vi "A170316-11_Auto.vi"() -> ()   [LabVIEW 2020]
uses:
  Global_Variable/A170316-11.vi
  Global_Variable/Global.vi
  Database/Global1.vi
  <vilib>/addons/database/Connection.llb/DB Tools Open Connec (String).vi
  <vilib>/addons/database/NI_Database_API.lvlib
panel:
  out "请再次确认扭矩":bool
  in  "更换产品":refnum<vi>
  out "刻线涂色标":bool
  out "涂下传动轴螺栓色标":bool
  out "拆下辅具安装下轴固定螺栓并确认扭矩":bool
  in  "前序OK？":string
  out "主观判断是否合格":bool
  out "右转两圈检测":bool
  out "左转两圈检测":bool
  out "按启动按钮":bool
  out "涂下轴固定螺栓色标":bool
  out "安装下传动轴辅具螺栓并确认扭矩":bool
  out "请扫码":bool
  out "磨合次数":i32
  in  "判定结果":bool[][](array[boolean])=[[TRUE]]
  in  "STEP":string
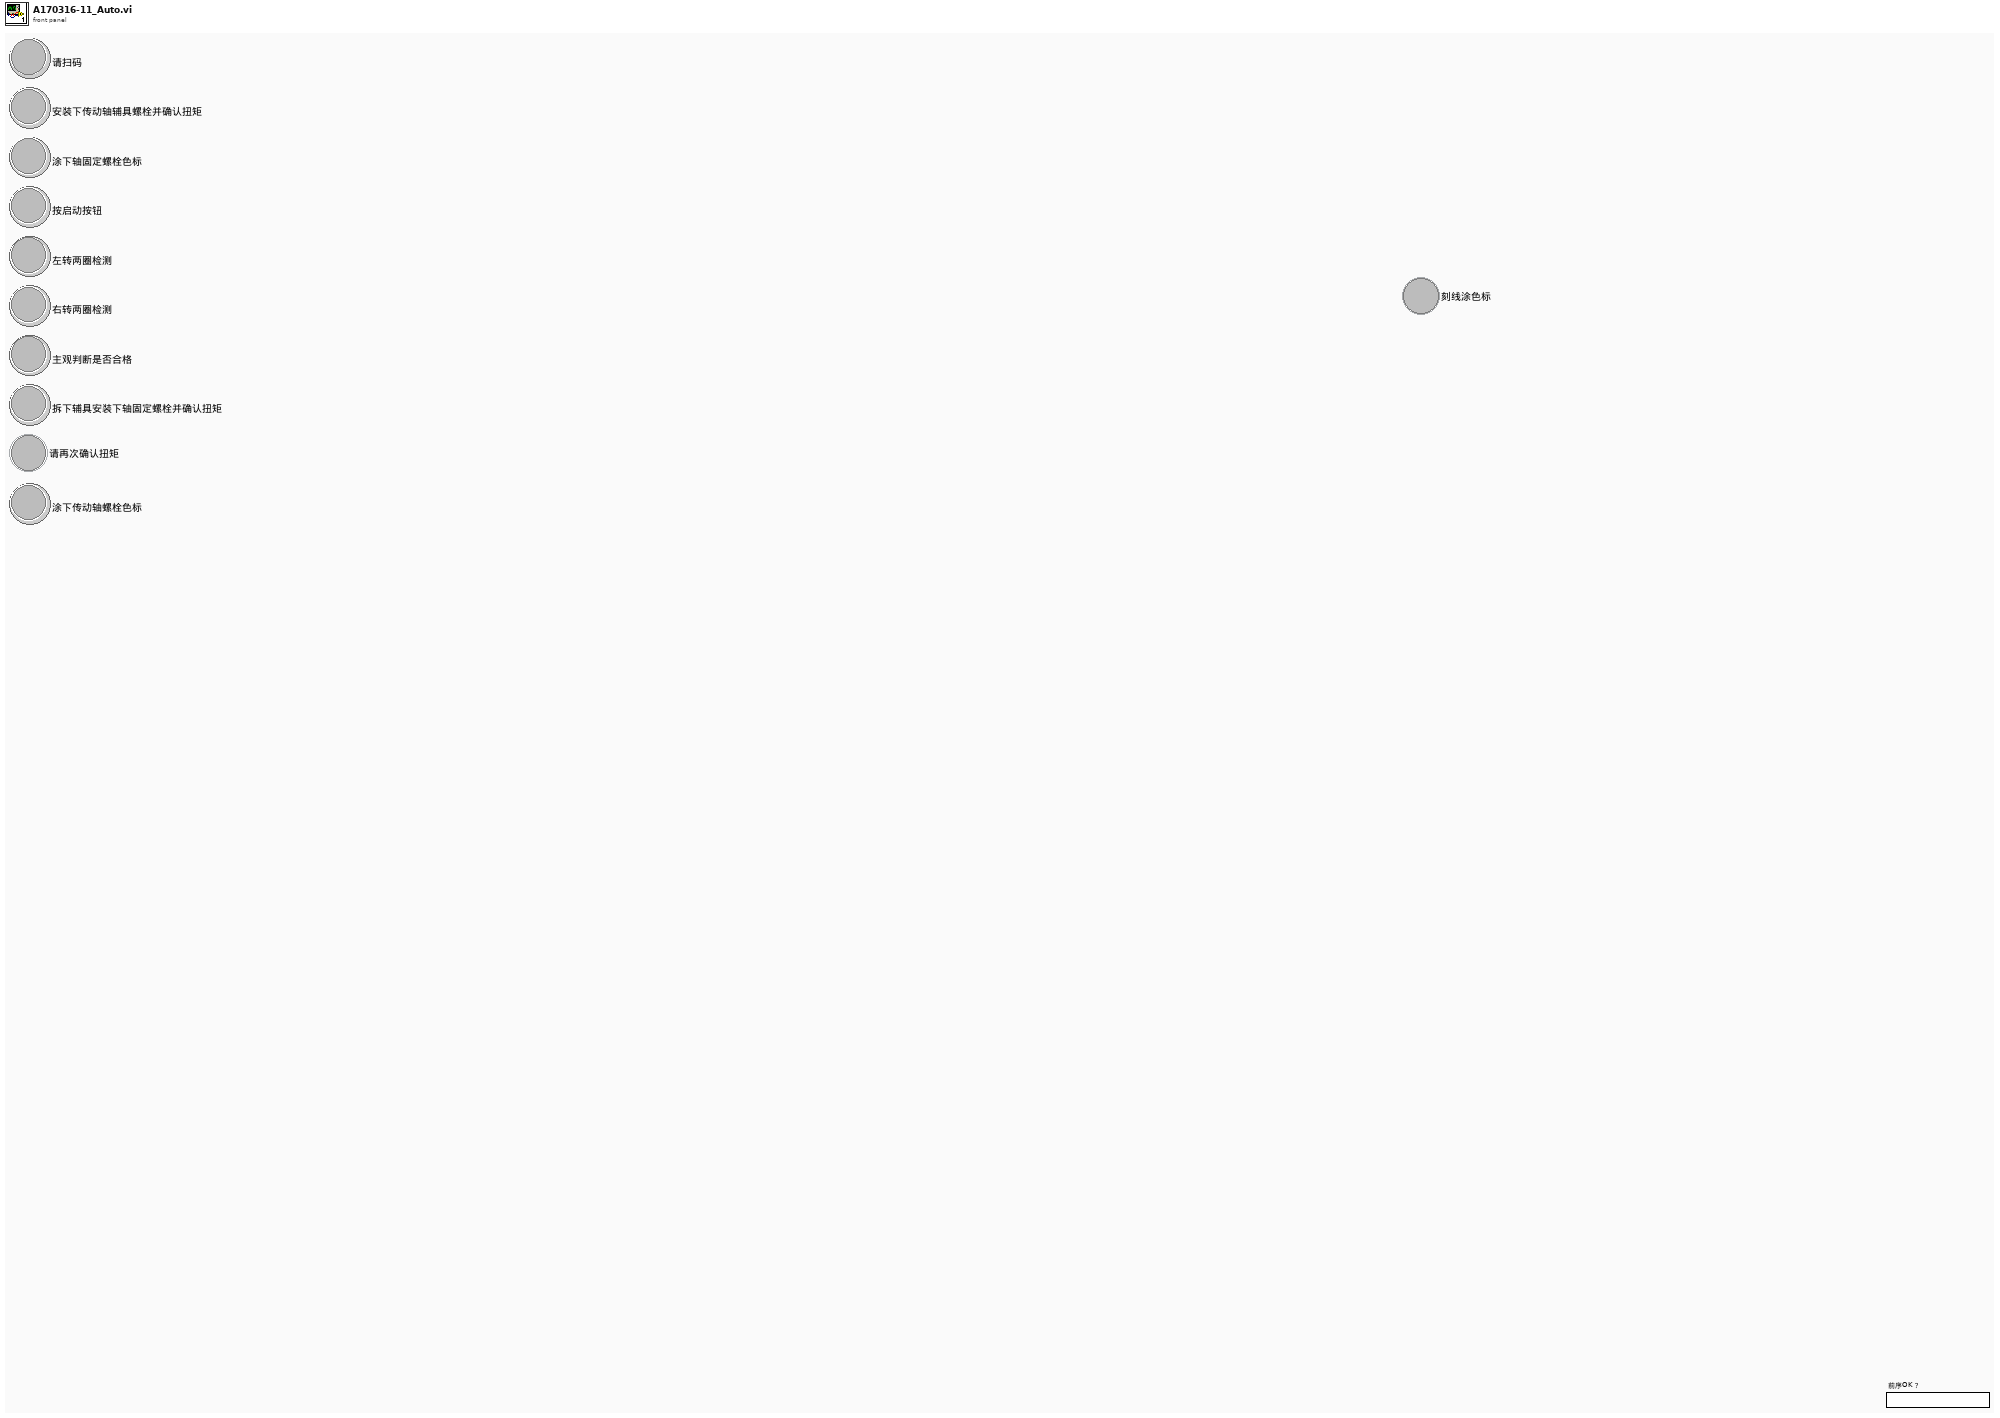
[diagram p1: front panel]
types:
  T1 = typedef "NI_Database_API.lvlib/Conn ObjectReference.ctl" = refnum<k1>
  T2 = cluster{i64, i64, i64, "生产结果":string, "result string":string}
  T3 = cluster{i64, i64, i64, "生产结果":string, "result string":string}[]
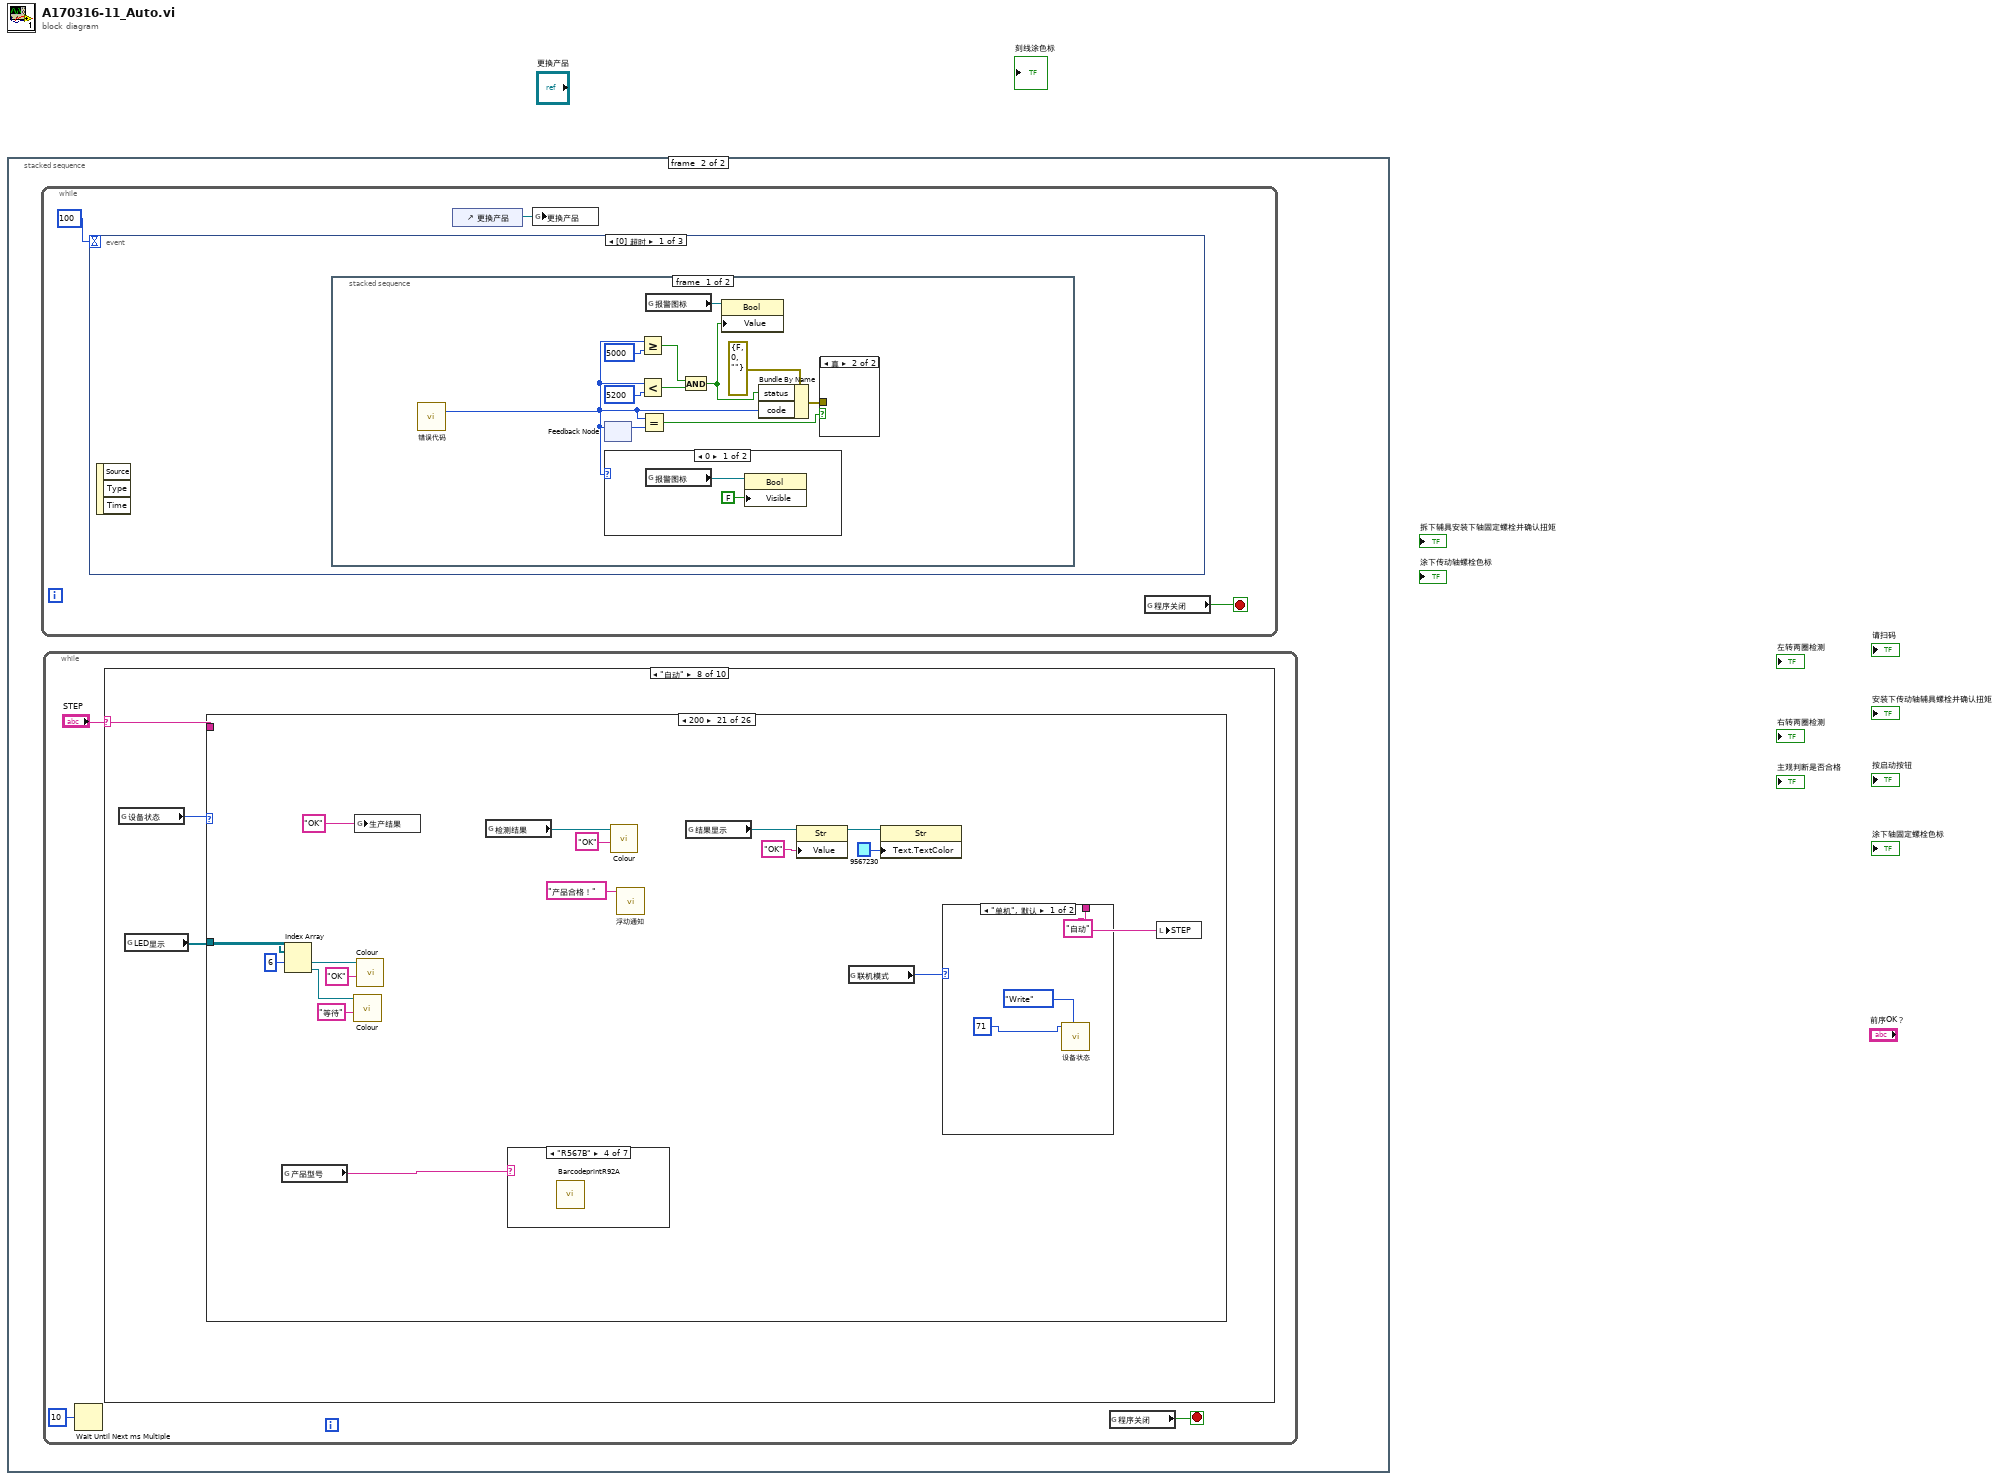
[diagram p0: block diagram]
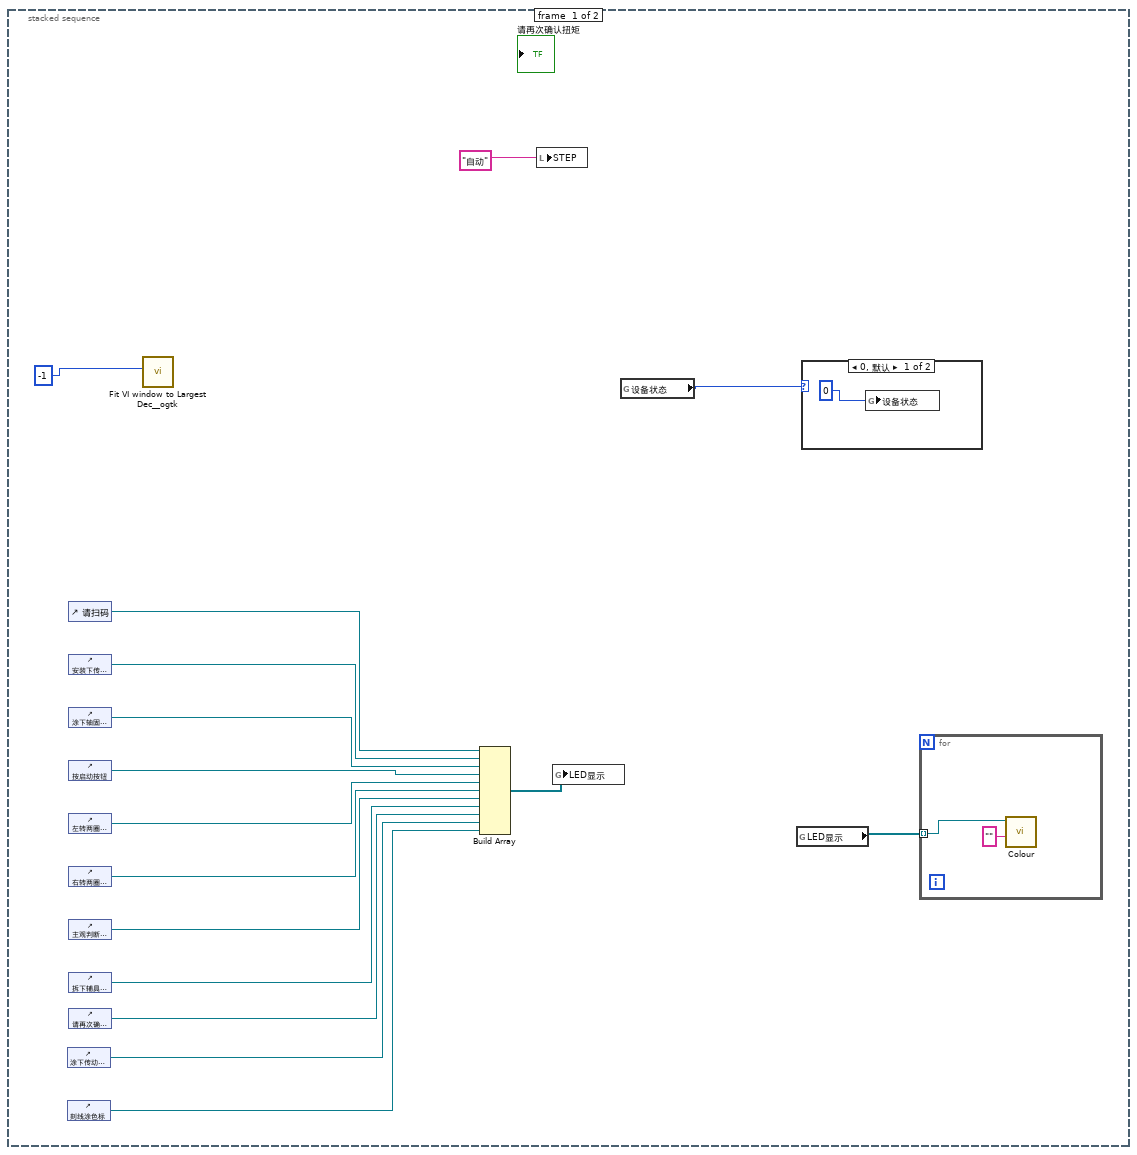
[diagram p2: hidden frame]
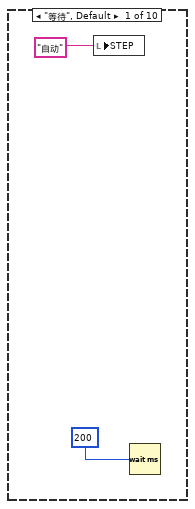
[diagram p4: hidden frame]
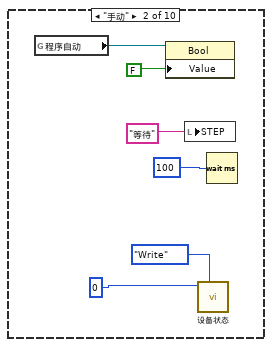
[diagram p5: hidden frame]
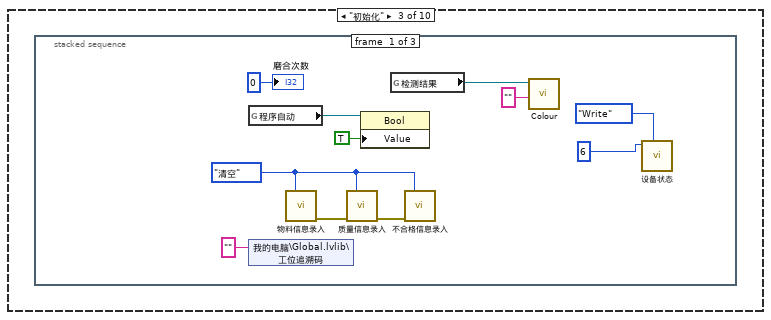
[diagram p6: hidden frame]
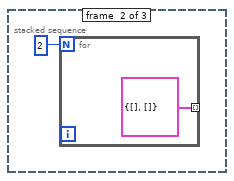
[diagram p7: hidden frame]
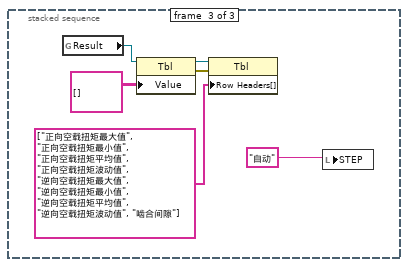
[diagram p8: hidden frame]
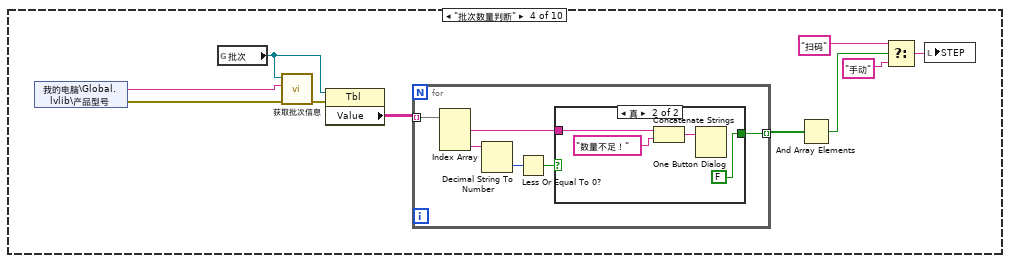
[diagram p9: hidden frame]
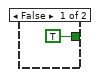
[diagram p10: hidden frame]
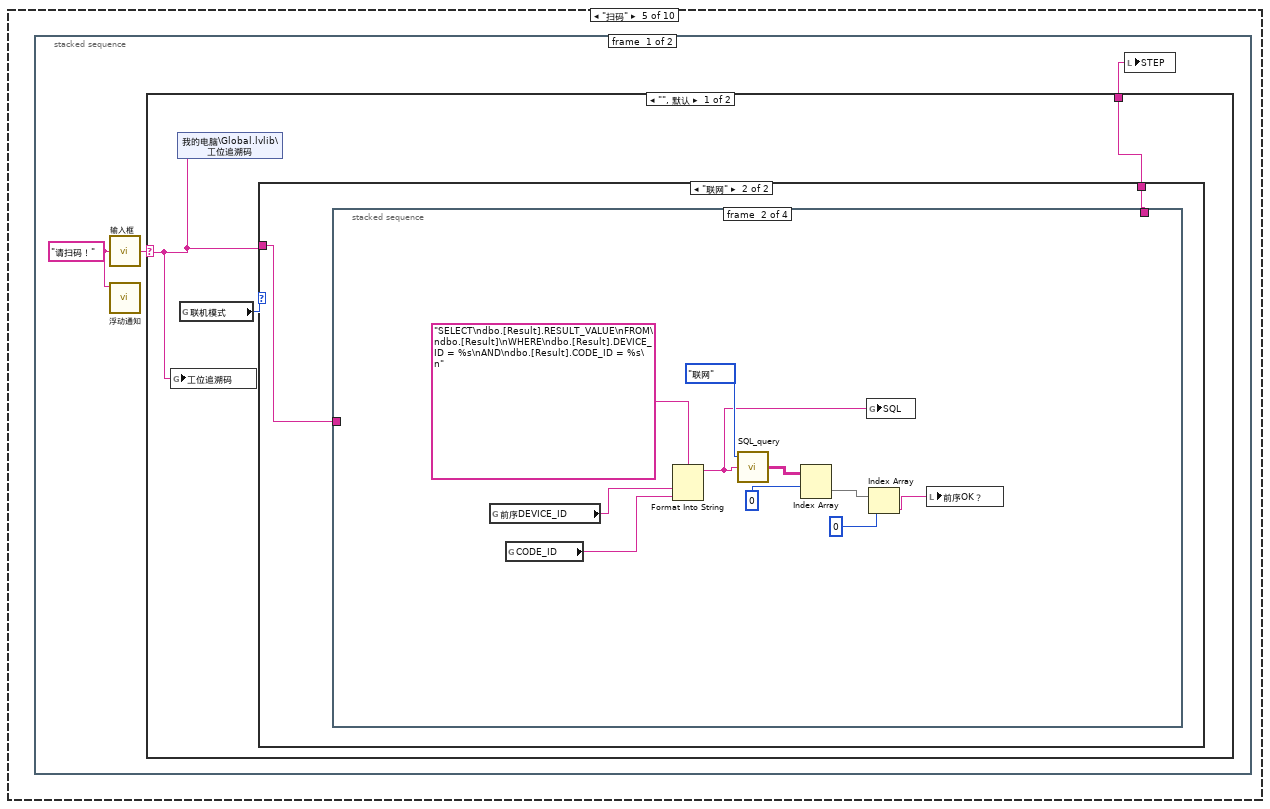
[diagram p11: hidden frame]
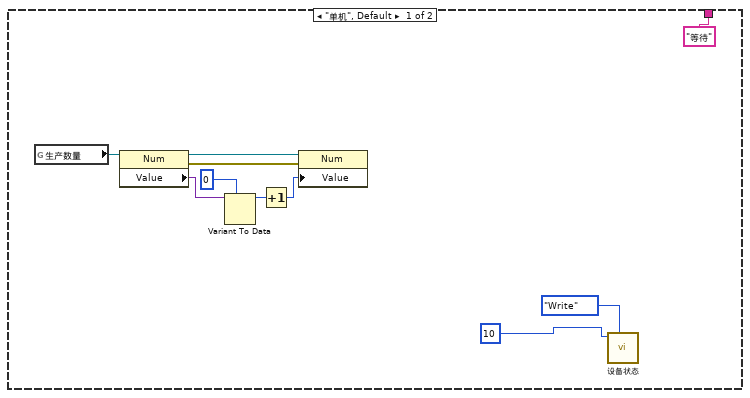
[diagram p12: hidden frame]
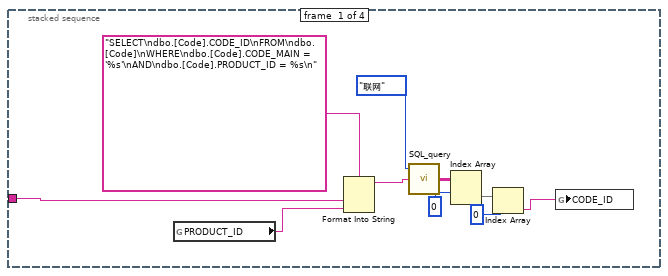
[diagram p13: hidden frame]
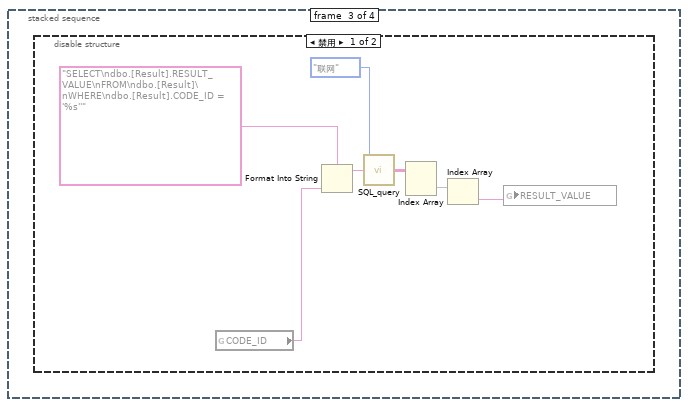
[diagram p14: hidden frame]
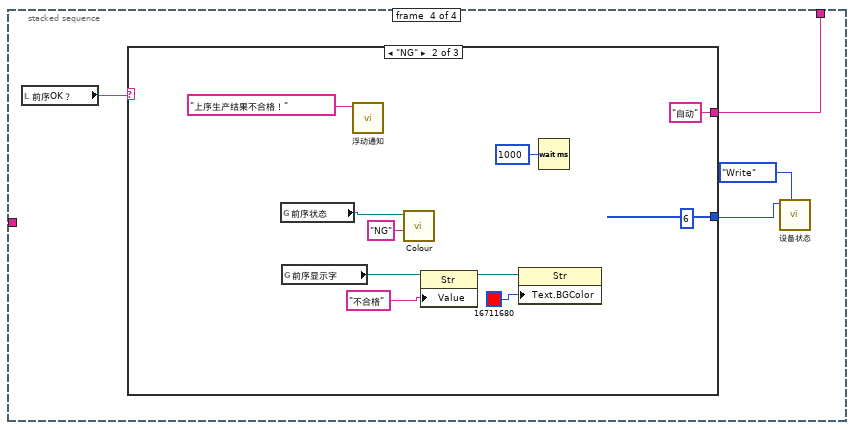
[diagram p16: hidden frame]
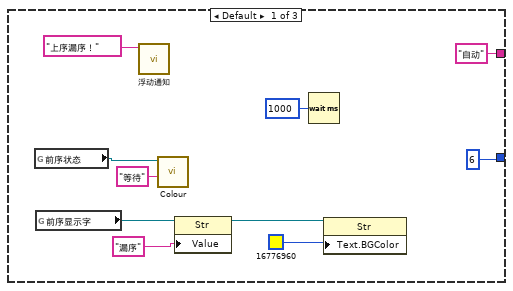
[diagram p17: hidden frame]
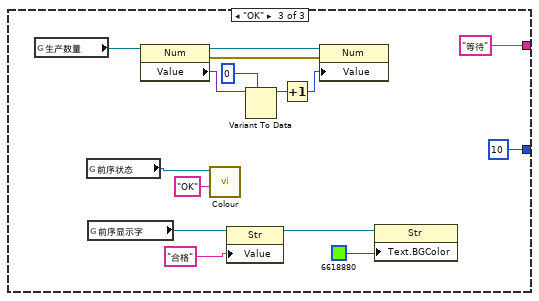
[diagram p18: hidden frame]
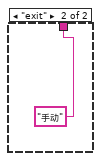
[diagram p19: hidden frame]
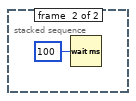
[diagram p20: hidden frame]
diagram:
  n1 = stacked-sequence {
    frame #0 {
      n2 = control-ref of="涂下传动轴螺栓色标"() -> (w4:refnum<vi>)
      n3 = control-ref of="刻线涂色标"() -> (w3:refnum<vi>)
      n4 = control-ref of="请扫码"() -> (w14:refnum<vi>)
      n5 = control-ref of="安装下传动轴辅具螺栓并确认扭矩"() -> (w13:refnum<vi>)
      n6 = control-ref of="涂下轴固定螺栓色标"() -> (w12:refnum<vi>)
      n7 = control-ref of="按启动按钮"() -> (w11:refnum<vi>)
      n8 = control-ref of="左转两圈检测"() -> (w10:refnum<vi>)
      n9 = control-ref of="右转两圈检测"() -> (w9:refnum<vi>)
      n10 = control-ref of="主观判断是否合格"() -> (w8:refnum<vi>)
      n11 = control-ref of="拆下辅具安装下轴固定螺栓并确认扭矩"() -> (w5:refnum<vi>)
      n12 = control-ref of="请再次确认扭矩"() -> (w2:refnum<vi>)
      n13 = call <userlib>:"Fit VI window to Largest Dec__ogtk.vi"("border spacing (2 px)"=-1) -> ()  [unwired: 5 in, 2 out]
      n14 = Build Array(w14, w13, w12, w11, w10, w9, w8, w5, w2, w4, w3) -> (w7:refnum<vi>[])
      n15 = local write "STEP"("自动" ("STEP")) -> ()
      n16 = global write "A170316-11.vi" "LED显示"(w7) -> ()
      n17 = global read "Global.vi" "设备状态"() -> (w1:i32)
      n18 = global read "A170316-11.vi" "LED显示"() -> (w6:refnum<vi>[])
      n19 = case shown="0, 默认" w1 {
        frame 0, Default {
          n20 = global write "Global.vi" "设备状态"(i16 0 ("设备状态")) -> ()
        }
        frame 3721..3723 {
        }
      }
      n21 = for {
        tunnel: w6 -> [w19] mode=indexing
        n22 = call "Colour.vi"("result"="", "colourRef"=w19) -> ()  [unwired: 9 in, 1 out]
      }
    }
    frame #1 {
      n23 = while {
        stop <- w463 stop-if-true
        n24 = event shown="[0] 超时" {
          selector: _ -> [_ _ _]
          dyn-events: _ -> [_ _ _]
          timeout: 100 -> [_ _ _]
          event Timeout {
            n25 = event-data() -> ()  [unwired: 1 in, 3 out]
            n26 = stacked-sequence {
              frame #0 {
                n27 = call "错误代码.vi"() -> ("Status_Read"=w465:u32)  [unwired: 11 in]
                n28 = feedback #1() -> (w475:u32)  [unwired: 1 in]
                n29 = feedback-in #1(w465) -> ()
                n30 = case shown="0" w465 {
                  frame 0 {
                    n31 = global read "Global.vi" "报警图标"() -> (w476:refnum<vi>)
                    n32 = property class="Bool"(reference=w476, "Visible"=FALSE ("可见")) -> ()  [unwired: 1 in, 2 out]
                  }
                  frame 1, Default {
                    n33 = global read "Global.vi" "报警图标"() -> (w479:refnum<vi>)
                    n34 = property class="Bool"(reference=w479, "Visible"=TRUE ("可见")) -> ()  [unwired: 1 in, 2 out]
                  }
                }
                n35 = Greater Or Equal?(x=w465, y=i16 5000) -> (x >= y?=w473:bool)
                n36 = Less?(x=w465, y=i16 5200) -> (x < y?=w474:bool)
                n37 = Equal?(x=w465, y=w475) -> (x = y?=w472:bool)
                n38 = global read "Global.vi" "报警图标"() -> (w467:refnum<vi>)
                n39 = And(x=w473, y=w474) -> (x .and. y?=w466:bool)
                n40 = property class="Bool"(reference=w467, "Value"=w466) -> ()  [unwired: 1 in, 2 out]
                n41 = Bundle By Name(cluster=errorcluster {"status"=FALSE, "code"=0, "source"=""} ("错误常量"), "status"=w466, "code"=w465) -> (w471:errorcluster)
                n42 = case shown="真" w472 {
                  tunnel: w471 -> [w480 _]
                  frame False {
                    n43 = call "报警处理.vi"("错误常量"=w480) -> ()  [unwired: 9 in, 2 out]
                  }
                  frame True {
                  }
                }
              }
              frame #1 {
                n44 = disable-structure shown="禁用" {
                  frame Disabled {
                    n45 = global read "Global.vi" "程序自动"() -> (w484:refnum<vi>)
                    n46 = property class="Bool"(reference=w484) -> ("Value"=w483:variant)  [unwired: 1 in, 2 out]
                    n47 = Variant To Data(type=FALSE, Variant=w483) -> (data=w481:bool)  [unwired: 1 in, 1 out]
                    n48 = case shown="真" w481 {
                      selector: w481 -> [w486 _]
                      frame False {
                        n49 = call <userlib>:"Boolean Trigger__ogtk.vi"("Boolean Input"=w486) -> ("Rising Edge"=w485:bool)  [unwired: 1 in, 1 out]
                        n50 = case shown="真" w485 {
                          frame False {
                          }
                          frame True {
                            n51 = local write "STEP"("手动" ("STEP")) -> ()
                          }
                        }
                      }
                      frame True {
                        n52 = shared-variable "我的电脑\\A17031611.lvlib\\设备状态"() -> (w488:i16)  [unwired: 1 in, 1 out]
                        n53 = case shown="5" w488 {
                          frame 0, Default {
                            n54 = global read "Global.vi" "程序自动"() -> (w490:refnum<vi>)
                            n55 = call "浮动通知.vi"("通知内容"="请复位") -> ()  [unwired: 11 in]
                            n56 = property class="Bool"(reference=w490, "Value"=FALSE) -> ()  [unwired: 1 in, 2 out]
                          }
                          frame 5 {
                            n57 = local write "STEP"("初始化" ("STEP")) -> ()
                          }
                        }
                      }
                    }
                  }
                  frame Enabled {
                  }
                }
              }
            }
          }
          event "更换产品": Value Change {
            n58 = event-data() -> ()  [unwired: 1 in, 6 out]
            n59 = global read "A170316-11.vi" "LED显示"() -> (w495:refnum<vi>[])
            n60 = global read "Global.vi" "操作步骤"() -> (w493:bool[])
            n61 = for "For循环" {
              tunnel: w493 -> [w499] mode=indexing
              tunnel: w495 -> [w498] mode=indexing
              shift-right: [w496] -> _
              shift-left: 360 -> [w497]
              n62 = case shown="真" w499 {
                tunnel: w498 -> [w501 w503]
                tunnel: w497 -> [w502 w508]
                tunnel: [w502 w505] -> w496
                frame False {
                  n63 = property class="Bool (严格)"(reference=w501, "Top"=-100 ("位置:置顶")) -> ()  [unwired: 1 in, 2 out]
                }
                frame True {
                  n64 = Add(x=w508, y=65) -> (x+y=w505:i32)
                  n65 = Bundle(-1510, w505) -> (w506:cluster{i32, i32})  [unwired: 1 in]
                  n66 = property class="Bool (严格)"(reference=w503, "Position"=w506) -> ()  [unwired: 1 in, 2 out]
                }
              }
            }
          }
          event Panel Close {
            n67 = event-data() -> ()  [unwired: 1 in, 4 out]
            n68 = global write "Global.vi" "程序关闭"(TRUE ("程序关闭")) -> ()
          }
        }
        n69 = control-ref of="更换产品"() -> (w462:refnum<vi>)
        n70 = global write "Global.vi" "更换产品"(w462) -> ()
        n71 = global read "Global.vi" "程序关闭"() -> (w463:bool)
      }
      n72 = while {
        stop <- w21 stop-if-true
        n73 = Wait Until Next ms Multiple(millisecond multiple=u32 10 ("毫秒倍数")) -> ()  [unwired: 1 out]
        n74 = case shown="\"自动\"" "STEP" {
          selector: "STEP" -> [_ _ _ _ _ _ _ w248 _ _]
          frame "等待", Default {
            n75 = local write "STEP"("自动" ("STEP")) -> ()
            n76 = Wait (ms)(milliseconds to wait=u32 200 ("等待时间（毫秒）")) -> ()  [unwired: 1 out]
          }
          frame "手动" {
            n77 = global read "Global.vi" "程序自动"() -> (w28:refnum<vi>)
            n78 = property class="Bool"(reference=w28, "Value"=FALSE) -> ()  [unwired: 1 in, 2 out]
            n79 = local write "STEP"("等待" ("STEP")) -> ()
            n80 = call "设备状态.vi"("枚举"=enum16{"Read", "Write"}."Write", "Status_Write"=u16 0 ("设备状态")) -> ()  [unwired: 9 in, 1 out]
            n81 = Wait (ms)(milliseconds to wait=u32 100 ("等待时间（毫秒）")) -> ()  [unwired: 1 out]
          }
          frame "初始化" {
            n82 = stacked-sequence {
              frame #0 {
                w40 = enum16{"录入", "清空"}."清空" ("功能")
                n83 = global read "Global.vi" "程序自动"() -> (w36:refnum<vi>)
                n84 = shared-variable "我的电脑\\Global.lvlib\\工位追溯码"("" ("传感器码")) -> ()  [unwired: 1 in, 1 out]
                n85 = call "物料信息录入.vi"("功能"=w40) -> ("错误输出"=w39:errorcluster)  [unwired: 14 in]
                n86 = call "质量信息录入.vi"("功能"=w40, "错误输入（无错误）"=w39) -> ("错误输出"=w41:errorcluster)  [unwired: 13 in]
                n87 = property class="Bool"(reference=w36, "Value"=TRUE) -> ()  [unwired: 1 in, 2 out]
                n88 = global read "Global.vi" "检测结果"() -> (w34:refnum<vi>)
                n89 = call "不合格信息录入.vi"("功能"=w40, "错误输入（无错误）"=w41) -> ()  [unwired: 13 in, 1 out]
                n90 = call "Colour.vi"("result"="", "colourRef"=w34) -> ()  [unwired: 9 in, 1 out]
                n91 = call "设备状态.vi"("枚举"=enum16{"Read", "Write"}."Write", "Status_Write"=i16 6 ("设备状态")) -> ()  [unwired: 9 in, 1 out]
                "磨合次数" <- 0 ("磨合次数")
              }
              frame #1 {
                n92 = for {
                  N: 2 -> [_]
                  tunnel: [cluster{dbl[], dbl[]} {[], []}] -> _ mode=indexing
                }
              }
              frame #2 {
                n93 = global read "Global.vi" "Result"() -> (w47:refnum<vi>)
                n94 = property class="Tbl"(reference=w47, "Value"=string[][] []) -> (reference out=w48:refnum<vi>, error out=w49:errorcluster)  [unwired: 1 in]
                n95 = property class="Tbl"(reference=w48, error in=w49, "Row Headers[]"=string[] ["正向空载扭矩最大值", "正向空载扭矩最小值", "正向空载扭矩平均值", "正向空载扭矩波动值", "逆向空载扭矩最大值", "逆向空载扭矩最小值", "逆向空载扭矩平均值", "逆向空载扭矩波动值", "啮合间隙"] ("列首字符串[]")) -> ()  [unwired: 2 out]
                n96 = local write "STEP"("自动" ("result")) -> ()
              }
            }
          }
          frame "批次数量判断" {
            n97 = shared-variable "我的电脑\\Global.lvlib\\产品型号"() -> (w55:string, error out=w58:errorcluster)  [unwired: 1 in]
            n98 = global read "Global.vi" "批次"() -> (w56:refnum<vi>)
            n99 = call "获取批次信息.vi"("error in (no error)"=w58, "产品型号"=w55, "Tbl引用句柄"=w56) -> ("error out"=w57:errorcluster)  [unwired: 7 in, 1 out]
            n100 = property class="Tbl"(reference=w56, error in=w57) -> ("Value"=w59:string[][])  [unwired: 2 out]
            n101 = for {
              tunnel: w59 -> [w65] mode=indexing
              tunnel: [w60] -> w54 mode=indexing
              n102 = Index Array(array=w65) -> (element #1=w61:string, element #3=w64:string)  [unwired: 3 in, 1 out]
              n103 = Decimal String To Number(string=w64) -> (number=w63:i32)  [unwired: 2 in, 1 out]
              n104 = Less Or Equal To 0?(x=w63) -> (x <= 0?=w62:bool)
              n105 = case shown="真" w62 {
                tunnel: w61 -> [_ w70]
                tunnel: [TRUE FALSE] -> w60
                frame False {
                }
                frame True {
                  n106 = Concatenate Strings(w70, "数量不足！" ("字符串")) -> (w68:string)
                  n107 = One Button Dialog(message=w68) -> ()  [unwired: 1 in, 1 out]
                }
              }
            }
            n108 = And Array Elements(Boolean array=w54) -> (logical AND=w53:bool)
            n109 = Select(t="扫码" ("STEP"), s=w53, f="手动" ("STEP")) -> (s? t:f=w50:string)
            n110 = local write "STEP"(w50) -> ()
          }
          frame "扫码" {
            n111 = stacked-sequence {
              frame #0 {
                w72 = "请扫码！" ("提示信息")
                n112 = call "输入框.vi"("提示信息"=w72) -> ("条形码输出"=w73:string)
                n113 = call "浮动通知.vi"("通知内容"=w72) -> ()  [unwired: 11 in]
                n114 = case shown="\"\", 默认" w73 {
                  selector: w73 -> [w74 _]
                  tunnel: [w75 "手动"] -> w71
                  frame "", Default {
                    n115 = global write "Global1.vi" "工位追溯码"(w74) -> ()
                    n116 = shared-variable "我的电脑\\Global.lvlib\\工位追溯码"(w74) -> ()  [unwired: 1 in, 1 out]
                    n117 = global read "Global1.vi" "联机模式"() -> (w76:enum16{"单机", "联网"})
                    n118 = case shown="\"联网\"" w76 {
                      tunnel: w74 -> [_ w87]
                      tunnel: ["等待" w88] -> w75
                      frame "单机", Default {
                        n119 = global read "Global.vi" "生产数量"() -> (w81:refnum<vi>)
                        n120 = property class="Num"(reference=w81) -> (reference out=w82:refnum<vi>, error out=w83:errorcluster, "Value"=w84:variant)  [unwired: 1 in]
                        n121 = Variant To Data(type=u32 0, Variant=w84) -> (data=w85:u32)  [unwired: 1 in, 1 out]
                        n122 = Increment(x=w85) -> (x+1=w86:u32)
                        n123 = property class="Num"(reference=w82, error in=w83, "Value"=w86) -> ()  [unwired: 2 out]
                        n124 = call "设备状态.vi"("枚举"=enum16{"Read", "Write"}."Write", "Status_Write"=i16 10 ("设备状态控制字")) -> ()  [unwired: 9 in, 1 out]
                      }
                      frame "联网" {
                        n125 = stacked-sequence {
                          tunnel: w87 -> [w95 _ _ _]
                          tunnel: [_ _ _ w119] -> w88
                          frame #0 {
                            n126 = global read "Global1.vi" "PRODUCT_ID"() -> (w92:string)
                            n127 = Format Into String(format string="SELECT\ndbo.[Code].CODE_ID\nFROM\ndbo.[Code]\nWHERE\ndbo.[Code].CODE_MAIN = '%s'\nAND\ndbo.[Code].PRODUCT_ID = %s\n" ("格式字符串"), w95, w92) -> (resulting string=w94:string)  [unwired: 2 in, 1 out]
                            n128 = call "SQL_query.vi"("SQL query"=w94, "联机模式"=enum16{"单机", "联网"}."联网") -> ("data"=w98:string[][])  [unwired: 1 in, 2 out]
                            n129 = Index Array(array=w98, index (row)=0 ("索引 (行)")) -> (element=w97:string[])  [unwired: 1 in]
                            n130 = Index Array(array=w97, index=0 ("索引")) -> (element=w89:string)
                            n131 = global write "Global1.vi" "CODE_ID"(w89) -> ()
                          }
                          frame #1 {
                            n132 = global read "Global1.vi" "前序DEVICE_ID"() -> (w102:string)
                            n133 = global read "Global1.vi" "CODE_ID"() -> (w103:string)
                            n134 = Format Into String(format string="SELECT\ndbo.[Result].RESULT_VALUE\nFROM\ndbo.[Result]\nWHERE\ndbo.[Result].DEVICE_ID = %s\nAND\ndbo.[Result].CODE_ID = %s\n" ("格式字符串"), w102, w103) -> (resulting string=w99:string)  [unwired: 2 in, 1 out]
                            n135 = call "SQL_query.vi"("SQL query"=w99, "联机模式"=enum16{"单机", "联网"}."联网") -> ("data"=w108:string[][])  [unwired: 1 in, 2 out]
                            n136 = Index Array(array=w108, index (row)=0 ("索引 (行)")) -> (element=w100:string[])  [unwired: 1 in]
                            n137 = global write "Global1.vi" "SQL"(w99) -> ()
                            n138 = Index Array(array=w100, index=0 ("索引")) -> (element=w104:string)
                            n139 = local write "前序OK？"(w104) -> ()
                          }
                          frame #2 {
                            n140 = disable-structure shown="禁用" {
                              frame Disabled {
                                n141 = global read "Global1.vi" "CODE_ID"() -> (w110:string)
                                n142 = Format Into String(format string="SELECT\ndbo.[Result].RESULT_VALUE\nFROM\ndbo.[Result]\nWHERE\ndbo.[Result].CODE_ID = '%s''" ("格式字符串"), w110) -> (resulting string=w112:string)  [unwired: 2 in, 1 out]
                                n143 = call "SQL_query.vi"("SQL query"=w112, "联机模式"=enum16{"单机", "联网"}."联网") -> ("data"=w115:string[][])  [unwired: 1 in, 2 out]
                                n144 = Index Array(array=w115) -> (element=w113:string[])  [unwired: 2 in]
                                n145 = Index Array(array=w113) -> (element=w114:string)  [unwired: 1 in]
                                n146 = global write "Global1.vi" "RESULT_VALUE"(w114) -> ()
                              }
                              frame Enabled {
                              }
                            }
                          }
                          frame #3 {
                            n147 = local read "前序OK？"() -> (w118:string)
                            n148 = case shown="\"NG\"" w118 {
                              tunnel: [i16 6 ("设备状态控制字") i16 6 ("设备状态控制字") i16 10 ("设备状态控制字")] -> w117
                              tunnel: ["自动" "自动" "等待"] -> w119
                              frame Default {
                                n149 = global read "Global.vi" "前序状态"() -> (w125:refnum<vi>)
                                n150 = global read "Global.vi" "前序显示字"() -> (w126:refnum<vi>)
                                n151 = call "浮动通知.vi"("通知内容"="上序漏序！" ("Status")) -> ()  [unwired: 11 in]
                                n152 = call "Colour.vi"("result"="等待", "colourRef"=w125) -> ()  [unwired: 9 in, 1 out]
                                n153 = property class="Str"(reference=w126, "Value"="漏序" ("值")) -> (reference out=w122:refnum<vi>)  [unwired: 1 in, 1 out]
                                n154 = Wait (ms)(milliseconds to wait=u32 1000 ("等待时间（毫秒）")) -> ()  [unwired: 1 out]
                                n155 = property class="Str"(reference=w122, "Text.BGColor"=u32 16776960) -> ()  [unwired: 1 in, 2 out]
                              }
                              frame "NG" {
                                n156 = global read "Global.vi" "前序状态"() -> (w135:refnum<vi>)
                                n157 = global read "Global.vi" "前序显示字"() -> (w136:refnum<vi>)
                                n158 = call "浮动通知.vi"("通知内容"="上序生产结果不合格！" ("Status")) -> ()  [unwired: 11 in]
                                n159 = call "Colour.vi"("result"="NG", "colourRef"=w135) -> ()  [unwired: 9 in, 1 out]
                                n160 = property class="Str"(reference=w136, "Value"="不合格" ("值")) -> (reference out=w132:refnum<vi>)  [unwired: 1 in, 1 out]
                                n161 = property class="Str"(reference=w132, "Text.BGColor"=u32 16711680) -> ()  [unwired: 1 in, 2 out]
                                n162 = Wait (ms)(milliseconds to wait=u32 1000 ("等待时间（毫秒）")) -> ()  [unwired: 1 out]
                              }
                              frame "OK" {
                                n163 = global read "Global.vi" "生产数量"() -> (w152:refnum<vi>)
                                n164 = global read "Global.vi" "前序状态"() -> (w144:refnum<vi>)
                                n165 = global read "Global.vi" "前序显示字"() -> (w145:refnum<vi>)
                                n166 = property class="Num"(reference=w152) -> (reference out=w153:refnum<vi>, error out=w151:errorcluster, "Value"=w150:variant)  [unwired: 1 in]
                                n167 = call "Colour.vi"("result"="OK", "colourRef"=w144) -> ()  [unwired: 9 in, 1 out]
                                n168 = property class="Str"(reference=w145, "Value"="合格" ("值")) -> (reference out=w141:refnum<vi>)  [unwired: 1 in, 1 out]
                                n169 = Variant To Data(type=u32 0, Variant=w150) -> (data=w149:u32)  [unwired: 1 in, 1 out]
                                n170 = Increment(x=w149) -> (x+1=w148:u32)
                                n171 = property class="Num"(reference=w153, error in=w151, "Value"=w148) -> ()  [unwired: 2 out]
                                n172 = property class="Str"(reference=w141, "Text.BGColor"=u32 6618880) -> ()  [unwired: 1 in, 2 out]
                              }
                            }
                            n173 = call "设备状态.vi"("枚举"=enum16{"Read", "Write"}."Write", "Status_Write"=w117) -> ()  [unwired: 9 in, 1 out]
                          }
                        }
                      }
                    }
                  }
                  frame "exit" {
                  }
                }
                n174 = local write "STEP"(w71) -> ()
              }
              frame #1 {
                n175 = Wait (ms)(milliseconds to wait=u32 100 ("等待时间（毫秒）")) -> ()  [unwired: 1 out]
              }
            }
          }
          frame "录入数据库" {
            n176 = stacked-sequence {
              frame #0 {
                n177 = shared-variable "我的电脑\\Global.lvlib\\工位追溯码"() -> ()  [unwired: 1 in, 2 out]
                n178 = global read "Global1.vi" "工位追溯码"() -> (w157:string)
                n179 = global read "Global1.vi" "PRODUCT_ID"() -> (w161:string)
                n180 = Format Into String(format string="SELECT\ndbo.[Code].CODE_ID\nFROM\ndbo.[Code]\nWHERE\ndbo.[Code].CODE_MAIN = '%s'\nAND\ndbo.[Code].PRODUCT_ID = %s\n" ("格式字符串"), w157, w161) -> (resulting string=w163:string)  [unwired: 2 in, 1 out]
                n181 = call "SQL_query.vi"("SQL query"=w163, "联机模式"=enum16{"单机", "联网"}."联网") -> ("data"=w166:string[][])  [unwired: 1 in, 2 out]
                n182 = Index Array(array=w166, index (row)=0 ("索引 (行)")) -> (element=w165:string[])  [unwired: 1 in]
                n183 = Index Array(array=w165, index=0 ("索引")) -> (element=w158:string)
                n184 = global write "Global1.vi" "CODE_ID"(w158) -> ()
              }
              frame #1 {
                n185 = global read "Global1.vi" "CODE_ID"() -> (w168:string)
                n186 = Format Into String(format string="SELECT\ndbo.[Result].RESULT_VALUE\nFROM\ndbo.[Result]\nWHERE\ndbo.[Result].CODE_ID = %s" ("格式字符串"), w168) -> (resulting string=w170:string)  [unwired: 2 in, 1 out]
                n187 = call "SQL_query.vi"("SQL query"=w170, "联机模式"=enum16{"单机", "联网"}."联网") -> ("data"=w172:string[][])  [unwired: 1 in, 2 out]
                n188 = Index Array(array=w172) -> (element=w171:string[])  [unwired: 2 in]
                n189 = Index Array(array=w171) -> ()  [unwired: 1 in, 1 out]
              }
              frame #2 {
                n190 = Get Date/Time String(date format (0)=enum16{"short", "long", "abbreviated"}."short" ("日期格式(0)"), want seconds? (F)=FALSE ("需要秒？(F)")) -> (date string=w182:string, time string=w183:string)  [unwired: 1 in]
                n191 = global read "Global1.vi" "DEVICE_ID"() -> (w186:string)
                n192 = global read "Global1.vi" "USER_ID"() -> (w184:string)
                n193 = global read "Global1.vi" "CODE_ID"() -> (w185:string)
                n194 = global read "Global1.vi" "生产结果"() -> (w177:string)
                n195 = global read "Global1.vi" "联机模式"() -> (w193:enum16{"单机", "联网"})
                n196 = Concatenate Strings(w182, " " ("字符串"), w183) -> (w178:string)
                n197 = Decimal String To Number(string=w186, default (0L)=i64 0 ("默认(0 I32)")) -> (number=w175:i64)  [unwired: 1 in, 1 out]
                n198 = Decimal String To Number(string=w184, default (0L)=i64 0 ("默认(0 I32)")) -> (number=w174:i64)  [unwired: 1 in, 1 out]
                n199 = Decimal String To Number(string=w185, default (0L)=i64 0 ("默认(0 I32)")) -> (number=w173:i64)  [unwired: 1 in, 1 out]
                n200 = call "GetSQLstring.vi"("联机模式"=w193) -> ("错误输出"=w196:errorcluster, "连接字符串"=w195:string)  [unwired: 9 in]
                n201 = Search and Replace String(replace all?=TRUE ("替换全部？(F)"), input string=w178, search string="/" ("替换字符串(\"\")"), replace string="-" ("替换字符串(\"\")")) -> (result string=w176:string)  [unwired: 4 in, 3 out]
                n202 = call-poly <vilib>:"DB Tools Open Connection.vi"("error in (no error)"=w196, "connection information"=w195) -> ("error out"=w194:errorcluster, "connection reference"=w197:T1)  [unwired: 6 in]
                n203 = Bundle(w175, w174, w173, "生产结果"=w177, "result string"=w176) -> (w199:T2)  [unwired: 1 in]
                n204 = Build Array(w199) -> (w200:T3)
                n205 = for {
                  tunnel: w200 -> [w205] mode=indexing
                  tunnel: w197 -> [w203]
                  shift-right: [w201] -> w198
                  shift-left: w194 -> [w208]
                  w204 = string[] ["DEVICE_ID", "USER_ID", "CODE_ID", "RESULT_VALUE", "RESULT_TIME"] ("columns")
                  w206 = "Result" ("table")
                  n206 = call <vilib>:"DB Tools Insert Data.vi"("data"=w205, "error in (no error)"=w208, "columns"=w204, "table"=w206, "connection reference"=w203) -> ("error out"=w207:errorcluster, "connection reference out"=w202:T1)  [unwired: 5 in]
                  n207 = case shown="错误" w207 {
                    selector: w207 -> [w209 w230]
                    tunnel: w204 -> [_ w227]
                    tunnel: w202 -> [w210 w219]
                    tunnel: w206 -> [_ w231]
                    tunnel: w205 -> [_ w223]
                    tunnel: [w210 w218] -> _
                    tunnel: [w209 w217] -> w201
                    frame No Error {
                    }
                    frame Error {
                      n208 = Array Subset(array=w227, index=3 ("长度"), length=2 ("长度")) -> (w228:string[])
                      n209 = Unbundle(w223) -> (w212:i64, w215:i64, "生产结果"=w222:string, "result string"=w221:string)  [unwired: 1 out]
                      n210 = Number To Decimal String(number=w215) -> (decimal integer string=w216:string)  [unwired: 1 in]
                      n211 = Number To Decimal String(number=w212) -> (decimal integer string=w211:string)  [unwired: 1 in]
                      n212 = Concatenate Strings("WHERE CODE_ID =" ("condition"), w216, "AND DEVICE_ID = ", w211) -> (w224:string)
                      n213 = Bundle("生产结果"=w222, "result string"=w221) -> (w220:cluster{"生产结果":string, "result string":string})  [unwired: 1 in]
                      n214 = call <vilib>:"Clear Errors.vi"("error in (no error)"=w230) -> ("error out"=w229:errorcluster)  [unwired: 5 in, 1 out]
                      n215 = call <vilib>:"DB Tools Update Data.vi"("condition"=w224, "data"=w220, "error in (no error)"=w229, "columns"=w228, "table"=w231, "connection reference"=w219) -> ("error out"=w217:errorcluster, "connection reference out"=w218:T1)  [unwired: 4 in]
                    }
                  }
                }
                n216 = call <vilib>:"Simple Error Handler.vi"("error in (no error)"=w198) -> ()  [unwired: 4 in, 5 out]
              }
              frame #3 {
                n217 = call "浮动通知.vi"("通知内容"="数据录入成功！" ("Status")) -> ()  [unwired: 11 in]
                n218 = local write "STEP"("自动" ("STEP")) -> ()
                n219 = Wait (ms)(milliseconds to wait=u32 3000 ("等待时间（毫秒）")) -> ()  [unwired: 1 out]
                n220 = call "设备状态.vi"("枚举"=enum16{"Read", "Write"}."Write", "Status_Write"=i16 71 ("设备状态")) -> ()  [unwired: 9 in, 1 out]
              }
            }
          }
          frame "录入批次" {
            n221 = shared-variable "我的电脑\\Global.lvlib\\产品型号"() -> (w238:string)  [unwired: 1 in, 1 out]
            n222 = call "更新批次.vi"("型号"=w238) -> ("error out"=w239:errorcluster)  [unwired: 10 in]
            n223 = global read "Global.vi" "批次"() -> (w240:refnum<vi>)
            n224 = call "更新易损件.vi"("error in (no error)"=w239) -> ("error out"=w242:errorcluster)  [unwired: 10 in]
            n225 = property class="Tbl"(reference=w240, error in=w242) -> ("Value"=w241:string[][])  [unwired: 2 out]
            n226 = for {
              tunnel: w241 -> [w245] mode=indexing
              n227 = Index Array(array=w245) -> (element #1=w244:string, element #2=w243:string)  [unwired: 2 in]
              n228 = call "物料信息录入.vi"("物料名称"=w244, "功能"=enum16{"录入", "清空"}."录入", "物料编码"=w243) -> ()  [unwired: 12 in, 1 out]
            }
            n229 = local write "STEP"("等待" ("STEP")) -> ()
          }
          frame "自动" {
            n230 = global read "Global.vi" "设备状态"() -> (w247:i32)
            n231 = global read "A170316-11.vi" "LED显示"() -> (w249:refnum<vi>[])
            n232 = case shown="200" w247 {
              tunnel: w249 -> [_ _ _ w268 _ _ _ _ w297 w304 w313 w322 w331 w340 w350 w358 w367 w374 w382 _ w392 w413 _ _ _ _]
              tunnel: w248 -> [_ _ _ _ _ _ _ _ _ _ _ _ _ _ _ _ _ _ _ _ _ _ _ _ _ _]
              frame Default {
              }
              frame -128 {
                n233 = call "浮动通知.vi"("通知内容"="复位中……" ("Status")) -> ()  [unwired: 11 in]
                n234 = global read "Global.vi" "程序自动"() -> (w251:refnum<vi>)
                n235 = property class="Bool"(reference=w251, "Value"=FALSE) -> ()  [unwired: 1 in, 2 out]
              }
              frame 5 {
                n236 = call "浮动通知.vi"("通知内容"="复位完成" ("Status")) -> ()  [unwired: 11 in]
              }
              frame 6 {
                n237 = Index Array(array=w268, index #1=0 ("索引")) -> (element #1=w288:refnum<vi>, element #2=w287:refnum<vi>, element #3=w286:refnum<vi>, element #4=w285:refnum<vi>, element #5=w284:refnum<vi>, element #6=w283:refnum<vi>, element #7=w282:refnum<vi>, element #8=w261:refnum<vi>, element #9=w260:refnum<vi>, element #10=w258:refnum<vi>, element #11=w254:refnum<vi>)  [unwired: 10 in]
                n238 = call "Colour.vi"("result"="", "colourRef"=w260) -> ()  [unwired: 9 in, 1 out]
                n239 = call "Colour.vi"("result"="等待", "colourRef"=w288) -> ()  [unwired: 9 in, 1 out]
                n240 = call "Colour.vi"("result"="", "colourRef"=w287) -> ()  [unwired: 9 in, 1 out]
                n241 = call "Colour.vi"("result"="", "colourRef"=w286) -> ()  [unwired: 9 in, 1 out]
                n242 = call "Colour.vi"("result"="", "colourRef"=w285) -> ()  [unwired: 9 in, 1 out]
                n243 = call "Colour.vi"("result"="", "colourRef"=w284) -> ()  [unwired: 9 in, 1 out]
                n244 = call "Colour.vi"("result"="", "colourRef"=w283) -> ()  [unwired: 9 in, 1 out]
                n245 = call "Colour.vi"("result"="", "colourRef"=w282) -> ()  [unwired: 9 in, 1 out]
                n246 = call "Colour.vi"("result"="", "colourRef"=w261) -> ()  [unwired: 9 in, 1 out]
                n247 = call "Colour.vi"("result"="", "colourRef"=w258) -> ()  [unwired: 9 in, 1 out]
                n248 = call "Colour.vi"("result"="", "colourRef"=w254) -> ()  [unwired: 9 in, 1 out]
                n249 = global read "Global.vi" "结果显示"() -> (w272:refnum<vi>)
                n250 = global read "Global.vi" "前序显示字"() -> (w267:refnum<vi>)
                n251 = global read "Global.vi" "前序状态"() -> (w266:refnum<vi>)
                n252 = property class="Str"(reference=w272, "Value"="..." ("结果显示")) -> (reference out=w273:refnum<vi>)  [unwired: 1 in, 1 out]
                n253 = property class="Str"(reference=w267, "Value"="" ("值")) -> (reference out=w257:refnum<vi>)  [unwired: 1 in, 1 out]
                n254 = call "Colour.vi"("result"="", "colourRef"=w266) -> ()  [unwired: 9 in, 1 out]
                n255 = property class="Str"(reference=w273, "Text.TextColor"=u32 9567230) -> ()  [unwired: 1 in, 2 out]
                n256 = property class="Str"(reference=w257, "Text.BGColor"=u32 16777216 ("文本.文本颜色:背景色")) -> ()  [unwired: 1 in, 2 out]
                n257 = local write "STEP"("扫码" ("STEP")) -> ()
              }
              frame 0 {
                n258 = call "浮动通知.vi"("通知内容"="不在自动！" ("Status")) -> ()  [unwired: 11 in]
              }
              frame 7 {
                n259 = call "浮动通知.vi"("通知内容"="" ("Status")) -> ()  [unwired: 11 in]
              }
              frame 8 {
                n260 = call "浮动通知.vi"("通知内容"="程序停止！" ("Status")) -> ()  [unwired: 11 in]
              }
              frame 9 {
                n261 = call "浮动通知.vi"("通知内容"="套花键中" ("Status")) -> ()  [unwired: 11 in]
              }
              frame 10 {
                n262 = Index Array(array=w297, index #1=0 ("索引")) -> (element #1=w299:refnum<vi>, element #2=w295:refnum<vi>)  [unwired: 1 in]
                n263 = call "Colour.vi"("result"="OK", "colourRef"=w299) -> ()  [unwired: 9 in, 1 out]
                n264 = call "Colour.vi"("result"="等待", "colourRef"=w295) -> ()  [unwired: 9 in, 1 out]
                n265 = call "浮动通知.vi"("通知内容"="请安装下轴螺栓并确认扭矩！" ("Status")) -> ()  [unwired: 11 in]
                n266 = call "设备状态.vi"("枚举"=enum16{"Read", "Write"}."Write", "Status_Write"=i16 20 ("设备状态")) -> ()  [unwired: 9 in, 1 out]
              }
              frame 22 {
                n267 = Index Array(array=w304, index #1=1 ("索引")) -> (element #1=w310:refnum<vi>, element #2=w309:refnum<vi>)  [unwired: 1 in]
                n268 = call "浮动通知.vi"("通知内容"="请涂下轴固定螺栓色标！" ("Status")) -> ()  [unwired: 11 in]
                n269 = call "设备状态.vi"("枚举"=enum16{"Read", "Write"}."Write", "Status_Write"=i16 30 ("设备状态")) -> ()  [unwired: 9 in, 1 out]
                n270 = call "Colour.vi"("result"="OK", "colourRef"=w310) -> ()  [unwired: 9 in, 1 out]
                n271 = call "Colour.vi"("result"="等待", "colourRef"=w309) -> ()  [unwired: 9 in, 1 out]
              }
              frame 32 {
                n272 = Index Array(array=w313, index #1=2 ("索引")) -> (element #1=w318:refnum<vi>, element #2=w314:refnum<vi>)  [unwired: 1 in]
                n273 = call "浮动通知.vi"("通知内容"="请按启动按钮！" ("Status")) -> ()  [unwired: 11 in]
                n274 = call "设备状态.vi"("枚举"=enum16{"Read", "Write"}."Write", "Status_Write"=i16 40 ("设备状态")) -> ()  [unwired: 9 in, 1 out]
                n275 = call "Colour.vi"("result"="等待", "colourRef"=w314) -> ()  [unwired: 9 in, 1 out]
                n276 = call "Colour.vi"("result"="OK", "colourRef"=w318) -> ()  [unwired: 9 in, 1 out]
              }
              frame 42 {
                n277 = Index Array(array=w322, index #1=3 ("索引")) -> (element #1=w327:refnum<vi>, element #2=w323:refnum<vi>)  [unwired: 1 in]
                n278 = call "浮动通知.vi"("通知内容"="请向左转动两圈！" ("Status")) -> ()  [unwired: 11 in]
                n279 = call "设备状态.vi"("枚举"=enum16{"Read", "Write"}."Write", "Status_Write"=i16 50 ("设备状态")) -> ()  [unwired: 9 in, 1 out]
                n280 = call "Colour.vi"("result"="OK", "colourRef"=w327) -> ()  [unwired: 9 in, 1 out]
                n281 = call "Colour.vi"("result"="等待", "colourRef"=w323) -> ()  [unwired: 9 in, 1 out]
              }
              frame 52 {
                n282 = Index Array(array=w331, index #1=4 ("索引")) -> (element #1=w336:refnum<vi>, element #2=w332:refnum<vi>)  [unwired: 1 in]
                n283 = call "浮动通知.vi"("通知内容"="请向右转动两圈！" ("Status")) -> ()  [unwired: 11 in]
                n284 = call "设备状态.vi"("枚举"=enum16{"Read", "Write"}."Write", "Status_Write"=i16 60 ("设备状态")) -> ()  [unwired: 9 in, 1 out]
                n285 = call "Colour.vi"("result"="OK", "colourRef"=w336) -> ()  [unwired: 9 in, 1 out]
                n286 = call "Colour.vi"("result"="等待", "colourRef"=w332) -> ()  [unwired: 9 in, 1 out]
              }
              frame 62 {
                n287 = Index Array(array=w340, index #1=5 ("索引")) -> (element #1=w345:refnum<vi>, element #2=w341:refnum<vi>)  [unwired: 1 in]
                n288 = call "Colour.vi"("result"="等待", "colourRef"=w341) -> ()  [unwired: 9 in, 1 out]
                n289 = call "Colour.vi"("result"="OK", "colourRef"=w345) -> ()  [unwired: 9 in, 1 out]
                n290 = call "浮动通知.vi"("通知内容"="请判断是否合格！" ("Status")) -> ()  [unwired: 11 in]
                n291 = call "设备状态.vi"("枚举"=enum16{"Read", "Write"}."Write", "Status_Write"=i16 70 ("设备状态")) -> ()  [unwired: 9 in, 1 out]
              }
              frame 71 {
                n292 = Index Array(array=w350, index #1=7 ("索引")) -> (element #1=w352:refnum<vi>)  [unwired: 1 in, 1 out]
                n293 = call "Colour.vi"("result"="等待", "colourRef"=w352) -> ()  [unwired: 9 in, 1 out]
                n294 = call "浮动通知.vi"("通知内容"="拆掉下传动轴辅具，安装下传动轴！" ("Status")) -> ()  [unwired: 11 in]
                n295 = call "设备状态.vi"("枚举"=enum16{"Read", "Write"}."Write", "Status_Write"=i16 80 ("设备状态")) -> ()  [unwired: 9 in, 1 out]
              }
              frame 81 {
                n296 = Index Array(array=w358, index #1=7 ("索引")) -> (element #1=w361:refnum<vi>, element #2=w356:refnum<vi>)  [unwired: 1 in]
                n297 = call "Colour.vi"("result"="OK", "colourRef"=w361) -> ()  [unwired: 9 in, 1 out]
                n298 = call "Colour.vi"("result"="等待", "colourRef"=w356) -> ()  [unwired: 9 in, 1 out]
                n299 = call "浮动通知.vi"("通知内容"="请再次确认扭矩！" ("Status")) -> ()  [unwired: 11 in]
                n300 = call "设备状态.vi"("枚举"=enum16{"Read", "Write"}."Write", "Status_Write"=i16 82 ("设备状态")) -> ()  [unwired: 9 in, 1 out]
              }
              frame 83 {
                n301 = Index Array(array=w367, index #1=8 ("索引")) -> (element #1=w369:refnum<vi>, element #2=w365:refnum<vi>)  [unwired: 1 in]
                n302 = call "Colour.vi"("result"="OK", "colourRef"=w369) -> ()  [unwired: 9 in, 1 out]
                n303 = call "Colour.vi"("result"="等待", "colourRef"=w365) -> ()  [unwired: 9 in, 1 out]
                n304 = call "设备状态.vi"("枚举"=enum16{"Read", "Write"}."Write", "Status_Write"=i16 90 ("设备状态")) -> ()  [unwired: 9 in, 1 out]
              }
              frame 91 {
                n305 = Index Array(array=w374, index #1=9 ("索引")) -> (element #1=w378:refnum<vi>, element #2=w377:refnum<vi>)  [unwired: 1 in]
                n306 = call "Colour.vi"("result"="OK", "colourRef"=w378) -> ()  [unwired: 9 in, 1 out]
                n307 = call "Colour.vi"("result"="等待", "colourRef"=w377) -> ()  [unwired: 9 in, 1 out]
                n308 = call "设备状态.vi"("枚举"=enum16{"Read", "Write"}."Write", "Status_Write"=i16 92 ("设备状态")) -> ()  [unwired: 9 in, 1 out]
                n309 = call "浮动通知.vi"("通知内容"="刻线涂色标！" ("Status")) -> ()  [unwired: 11 in]
              }
              frame 93 {
                n310 = Index Array(array=w382, index #1=10 ("索引")) -> (element #1=w385:refnum<vi>)  [unwired: 1 in, 1 out]
                n311 = call "Colour.vi"("result"="OK", "colourRef"=w385) -> ()  [unwired: 9 in, 1 out]
                n312 = call "浮动通知.vi"("通知内容"="完成！" ("Status")) -> ()  [unwired: 11 in]
                n313 = call "设备状态.vi"("枚举"=enum16{"Read", "Write"}."Write", "Status_Write"=i16 94 ("设备状态")) -> ()  [unwired: 9 in, 1 out]
              }
              frame 101 {
                n314 = call "浮动通知.vi"("通知内容"="请放回检具10！" ("Status")) -> ()  [unwired: 11 in]
                n315 = call "设备状态.vi"("枚举"=enum16{"Read", "Write"}."Write", "Status_Write"=i16 103 ("设备状态")) -> ()  [unwired: 9 in, 1 out]
              }
              frame 200 {
                n316 = global read "Global.vi" "产品型号"() -> (w396:string)
                n317 = Index Array(array=w392, index #1=6 ("索引")) -> (element #1=w394:refnum<vi>, element #2=w390:refnum<vi>)  [unwired: 1 in]
                n318 = call "Colour.vi"("result"="等待", "colourRef"=w390) -> ()  [unwired: 9 in, 1 out]
                n319 = global write "Global1.vi" "生产结果"("OK" ("ECU工位生产结果")) -> ()
                n320 = call "Colour.vi"("result"="OK", "colourRef"=w394) -> ()  [unwired: 9 in, 1 out]
                n321 = global read "Global.vi" "检测结果"() -> (w406:refnum<vi>)
                n322 = case shown="\"R567B\"" w396 {
                  frame Default {
                    n323 = call "Barcodeprint.vi"() -> ()  [unwired: 12 in]
                  }
                  frame "R92A" {
                    n324 = call "BarcodeprintR92A.vi"() -> ()  [unwired: 12 in]
                  }
                  frame "R092B" {
                    n325 = call "BarcodeprintR92A.vi"() -> ()  [unwired: 12 in]
                  }
                  frame "R567B" {
                    n326 = call "BarcodeprintR92A.vi"() -> ()  [unwired: 12 in]
                  }
                  frame "R092C" {
                    n327 = call "BarcodeprintR92A.vi"() -> ()  [unwired: 12 in]
                  }
                  frame "R092D" {
                    n328 = call "BarcodeprintR92A.vi"() -> ()  [unwired: 12 in]
                  }
                  frame "R567D" {
                    n329 = call "BarcodeprintR92A.vi"() -> ()  [unwired: 12 in]
                  }
                }
                n330 = call "Colour.vi"("result"="OK", "colourRef"=w406) -> ()  [unwired: 9 in, 1 out]
                n331 = call "浮动通知.vi"("通知内容"="产品合格！" ("Status")) -> ()  [unwired: 11 in]
                n332 = global read "Global.vi" "结果显示"() -> (w404:refnum<vi>)
                n333 = property class="Str"(reference=w404, "Value"="OK" ("结果显示")) -> (reference out=w401:refnum<vi>)  [unwired: 1 in, 1 out]
                n334 = global read "Global1.vi" "联机模式"() -> (w397:enum16{"单机", "联网"})
                n335 = property class="Str"(reference=w401, "Text.TextColor"=u32 9567230) -> ()  [unwired: 1 in, 2 out]
                n336 = case shown="\"单机\", 默认" w397 {
                  tunnel: ["自动" "录入数据库"] -> w399
                  frame "单机", Default {
                    n337 = call "设备状态.vi"("枚举"=enum16{"Read", "Write"}."Write", "Status_Write"=i16 71 ("设备状态")) -> ()  [unwired: 9 in, 1 out]
                  }
                  frame "联网" {
                  }
                }
                n338 = local write "STEP"(w399) -> ()
              }
              frame 201 {
                n339 = global read "Global.vi" "检测结果"() -> (w426:refnum<vi>)
                n340 = Index Array(array=w413, index #1=6 ("索引")) -> (element #1=w415:refnum<vi>, element #2=w411:refnum<vi>)  [unwired: 1 in]
                n341 = global read "Global.vi" "产品型号"() -> (w420:string)
                n342 = call "Colour.vi"("result"="NG", "colourRef"=w415) -> ()  [unwired: 9 in, 1 out]
                n343 = call "Colour.vi"("result"="等待", "colourRef"=w411) -> ()  [unwired: 9 in, 1 out]
                n344 = call "Colour.vi"("result"="NG", "colourRef"=w426) -> ()  [unwired: 9 in, 1 out]
                n345 = case shown="默认" w420 {
                  frame Default {
                    n346 = call "Barcodeprint.vi"() -> ()  [unwired: 12 in]
                  }
                  frame "R92A" {
                    n347 = call "BarcodeprintR92A.vi"() -> ()  [unwired: 12 in]
                  }
                }
                n348 = global write "Global1.vi" "生产结果"("NG" ("ECU工位生产结果")) -> ()
                n349 = call "浮动通知.vi"("通知内容"="产品不合格！" ("Status")) -> ()  [unwired: 11 in]
                n350 = global read "Global1.vi" "联机模式"() -> (w418:enum16{"单机", "联网"})
                n351 = case shown="\"单机\", 默认" w418 {
                  tunnel: ["自动" "录入数据库"] -> w417
                  frame "单机", Default {
                    n352 = call "设备状态.vi"("枚举"=enum16{"Read", "Write"}."Write", "Status_Write"=i16 71 ("设备状态")) -> ()  [unwired: 9 in, 1 out]
                  }
                  frame "联网" {
                  }
                }
                n353 = global read "Global.vi" "结果显示"() -> (w425:refnum<vi>)
                n354 = property class="Str"(reference=w425, "Value"="NG" ("结果显示")) -> (reference out=w424:refnum<vi>)  [unwired: 1 in, 1 out]
                n355 = property class="Str"(reference=w424, "Text.TextColor"=u32 16711680) -> ()  [unwired: 1 in, 2 out]
                n356 = local write "STEP"(w417) -> ()
              }
              frame 1024 {
                n357 = call "浮动通知.vi"("通知内容"="急停！" ("Status")) -> ()  [unwired: 11 in]
                n358 = global read "Global.vi" "程序自动"() -> (w433:refnum<vi>)
                n359 = property class="Bool"(reference=w433, "Value"=FALSE) -> ()  [unwired: 1 in, 2 out]
              }
              frame 3721 {
                n360 = local write "STEP"("不合格锁定" ("STEP")) -> ()
                n361 = call "浮动通知.vi"("通知内容"="产品不合格程序锁定！" ("Status")) -> ()  [unwired: 11 in]
              }
              frame 3722 {
                n362 = global read "Global.vi" "程序自动"() -> (w438:refnum<vi>)
                n363 = call "浮动通知.vi"("通知内容"="授权成功，请复位！" ("Status")) -> ()  [unwired: 11 in]
                n364 = property class="Bool"(reference=w438, "Value"=FALSE) -> ()  [unwired: 1 in, 2 out]
              }
              frame 3723 {
                n365 = call "浮动通知.vi"("通知内容"="请取出不合格产品并摆放至不合格品区！" ("Status")) -> ()  [unwired: 11 in]
              }
            }
          }
          frame "不合格锁定" {
            n366 = call "临时授权.vi"() -> ("授权成功"=w442:bool)  [unwired: 11 in]
            n367 = case shown="真" w442 {
              frame False {
              }
              frame True {
                n368 = local write "STEP"("报表" ("STEP")) -> ()
                n369 = call "设备状态.vi"("枚举"=enum16{"Read", "Write"}."Write", "Status_Write"=i16 3722 ("设备状态")) -> ()  [unwired: 9 in, 1 out]
              }
            }
            n370 = Wait (ms)(milliseconds to wait=u32 100 ("等待时间（毫秒）")) -> ()  [unwired: 1 out]
          }
          frame "报表" {
            n371 = call "浮动通知.vi"("通知内容"="报表生成中" ("Status")) -> ()  [unwired: 11 in]
            n372 = Index Array(array="判定结果", index (col)=1 ("禁用的索引 (列)")) -> (element=w450:bool[])  [unwired: 1 in]
            n373 = And Array Elements(Boolean array=w450) -> (logical AND=w447:bool)
            n374 = shared-variable "我的电脑\\Global.lvlib\\联机模式"() -> (w452:i16)  [unwired: 1 in, 1 out]
            n375 = case shown="真" w447 {
              frame False {
              }
              frame True {
                n376 = global read "Global.vi" "合格数量"() -> (w461:refnum<vi>)
                n377 = property class="Num"(reference=w461) -> (reference out=w460:refnum<vi>, error out=w459:errorcluster, "Value"=w458:variant)  [unwired: 1 in]
                n378 = Variant To Data(type=u32 0, Variant=w458) -> (data=w457:u32)  [unwired: 1 in, 1 out]
                n379 = Increment(x=w457) -> (x+1=w456:u32)
                n380 = property class="Num"(reference=w460, error in=w459, "Value"=w456) -> ()  [unwired: 2 out]
              }
            }
            n381 = case shown="1" w452 {
              frame 0, Default {
              }
              frame 1 {
                n382 = call "上传数据库.vi"() -> ()  [unwired: 11 in, 1 out]
              }
            }
            n383 = global read "Global.vi" "设备状态"() -> (w446:i32)
            n384 = case shown="默认" w446 {
              frame Default {
                n385 = local write "STEP"("初始化" ("STEP")) -> ()
              }
              frame 3721..3723 {
                n386 = local write "STEP"("等待" ("STEP")) -> ()
              }
            }
          }
        }
        n387 = global read "Global.vi" "程序关闭"() -> (w21:bool)
      }
    }
  }
